vi "Configure Serial Output Data Rate.vi"(0 "fpga interface in":refnum<k20>, 5 "serial output channels":string[](array[string]), 7 "serial output data rates":dbl[](array[numeric])=[-1.0], 11 "error in (no error)":errorcluster) -> (4 "fpga interface out":refnum<k20>, 15 "error out":errorcluster)   [LabVIEW 2023, in "GettingStarted_Common_148X_Host.lvlib"]
uses:
  GettingStarted_Common_148X_Host.lvlib
  <instrlib>/FlexRIO/API/Host/v1/NI FlexRIO/API/Get Property Reference - Fpga Small.vi
  <resource>/objmgr/niflexrioapiChannel.rc
  <instrlib>/FlexRIO/API/Host/v1/NI FlexRIO API v1.lvlib
  <resource>/objmgr/niflexrioapi.rc
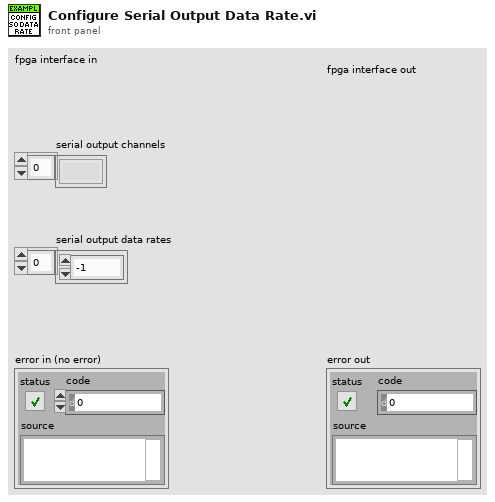
[diagram p1: front panel]
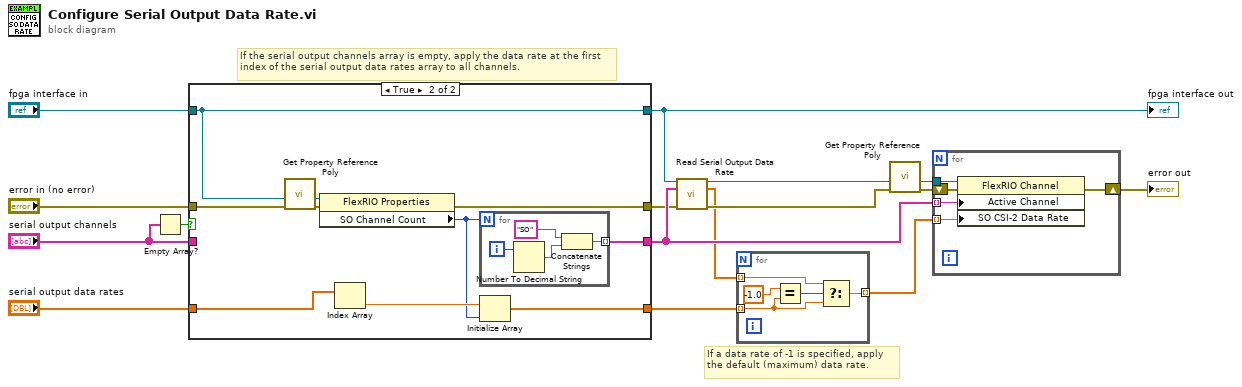
[diagram p0: block diagram]
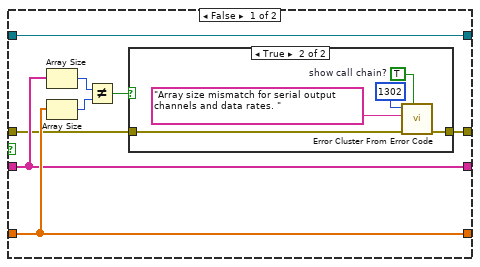
[diagram p2: hidden frame]
diagram:
  # "If a data rate of -1 is specified, apply the default (maximum) data rate."
  # "If the serial output channels array is empty, apply the data rate at the first index of the serial output data rates array to all channels."
  n1 = Empty Array?(array="serial output channels") -> (empty?=w10:bool)
  n2 = case shown="True" w10 {
    tunnel: "serial output channels" -> [w18 _]
    tunnel: "error in (no error)" -> [w17 w37]
    tunnel: [w18 w38] -> w13
    tunnel: "fpga interface in" -> [w24 w36]
    tunnel: [w24 w36] -> w6
    tunnel: [w20 w35] -> w5
    tunnel: "serial output data rates" -> [w19 w34]
    tunnel: [w19 w31] -> w2
    frame False {
      n3 = Array Size(array=w18) -> (size(s)=w22:i32)
      n4 = Array Size(array=w19) -> (size(s)=w23:i32)
      n5 = Not Equal?(x=w22, y=w23) -> (x != y?=w21:bool)
      n6 = case shown="True" w21 {
        tunnel: [w25 w26] -> w20
        tunnel: w17 -> [w25 w27]
        frame False {
        }
        frame True {
          w28 = TRUE  # show call chain?
          n7 = call <vilib>:"Error Cluster From Error Code.vi"("show call chain? (False)"=w28, "error in (no error)"=w27, "error message (\"\")"="Array size mismatch for serial output channels and data rates. ", "error code (0)"=1302) -> ("error out"=w26:errorcluster)  [unwired: 5 in]
        }
      }
    }
    frame True {
      n8 = call-poly <instrlib>:"Get Property Reference Poly.vi"("error in (no error)"=w37, "fpga interface in"=w36) -> ("error out"=w39:errorcluster, "property reference"=w40:refnum<k20>)  [unwired: 4 in, 1 out]
      n9 = property class="FlexRIO Properties"(reference=w40, error in=w39) -> (error out=w35:errorcluster, "SO Channel Count"=w32:i32)  [unwired: 1 out]
      n10 = Index Array(array=w34) -> (element=w33:dbl)  [unwired: 1 in]
      n11 = for {
        N: w32 -> [_]
        tunnel: [w41] -> w38 mode=indexing
        i -> [w44]
        n12 = Number To Decimal String(number=w44) -> (decimal integer string=w43:string)  [unwired: 1 in]
        n13 = Concatenate Strings("SO", w43) -> (w41:string)
      }
      n14 = Initialize Array(w33, w32) -> (w31:dbl[])
    }
  }
  "fpga interface out" <- w6
  n15 = call "Read Serial Output Data Rate.vi"("fpga interface in"=w6, "serial output channels"=w13, "error in (no error)"=w5) -> ("fpga interface out"=w12:refnum<k20>, "serial output data rates (bps)"=w3:dbl[], "error out"=w14:errorcluster)  [unwired: 10 in]
  n16 = for {
    tunnel: w3 -> [w46] mode=indexing
    tunnel: w2 -> [w48] mode=indexing
    tunnel: [w45] -> w1 mode=indexing
    n17 = Equal?(x=-1.0, y=w48) -> (x = y?=w49:bool)
    n18 = Select(t=w46, s=w49, f=w48) -> (s? t:f=w45:dbl)
  }
  n19 = call-poly <instrlib>:"Get Property Reference Poly.vi"("error in (no error)"=w14, "fpga interface in"=w12) -> ("error out"=w16:errorcluster, "property reference"=w15:refnum<k20>)  [unwired: 4 in, 1 out]
  n20 = for {
    tunnel: w15 -> [w53]
    tunnel: w1 -> [w52] mode=indexing
    tunnel: w13 -> [w51] mode=indexing
    shift-right: [w50] -> w11
    shift-left: w16 -> [w54]
    n21 = property class="FlexRIO Channel"(reference=w53, error in=w54, "Active Channel"=w51, "SO CSI-2 Data Rate"=w52) -> (error out=w50:errorcluster)  [unwired: 1 out]
  }
  "error out" <- w11
